vi "Log Data.vi"(8 "error in (no error)":errorcluster, 10 "Data Queue":refnum<queue>, 11 "Logging Configuration":T1={"Log Directory Path"=path "", "Log File Path"=path "", "Log File Prefix"="", "Log File Extension"="", "File Delimiter"=",", "Header Info"=[], "Channels"=[], "Log Instrument Runs"=FALSE}) -> (0 "error out":errorcluster)   [LabVIEW 2020, in "Mock Temperature Controller Control Panel.lvlib" / "Logging.lvlib"]
doc: "This VI uses the TDMS Write function to write data to a TDMS file."
uses:
  Logging.lvlib
  Logging Configuration.ctl
  Instrument Manager/Instrument State.ctl
  <vilib>/Utility/file.llb/Write Delimited Spreadsheet (string).vi
  Instrument Manager/Instrument Manager.lvlib
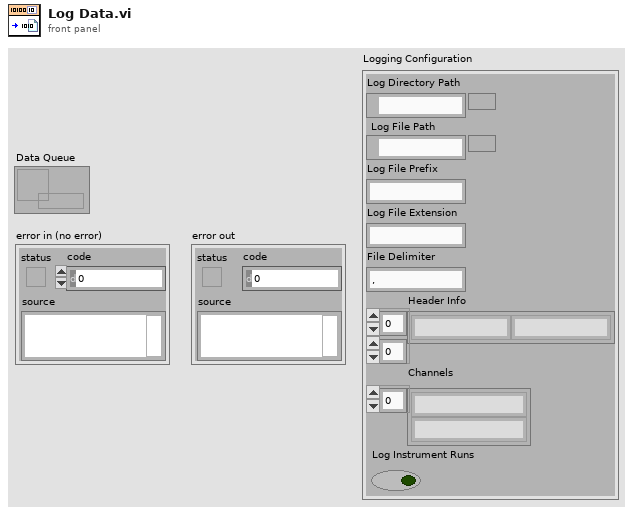
[diagram p1: front panel]
types:
  T1 = typedef "Mock Temperature Controller Control Panel.lvlib/Logging.lvlib/Logging Configuration.ctl" = cluster{"Log Directory Path":path, "Log File Path":path, "Log File Prefix":string, "Log File Extension":string, "File Delimiter":string, "Header Info":string[][], "Channels":string[], "Log Instrument Runs":bool}
  T2 = typedef "Mock Temperature Controller Control Panel.lvlib/Instrument Manager.lvlib/Instrument State.ctl" = cluster{"VISA Resource":refnum<visa-resource-name>, "Setpoint":dbl, "Running":bool, "Running Since":timestamp, "Data Point":cluster{"Time Stamp":timestamp, "Value":dbl}, "Current Temperature":dbl, "Sampling Rate (sec/sample)":dbl}
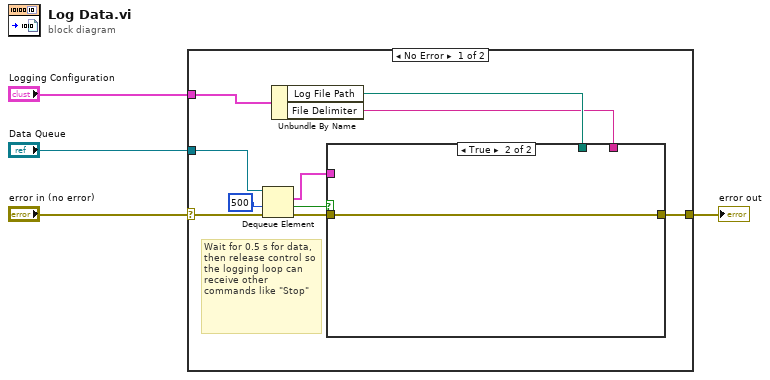
[diagram p0: block diagram]
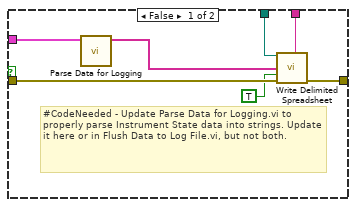
[diagram p2: hidden frame]
diagram:
  n1 = case shown="No Error" "error in (no error)" {
    selector: "error in (no error)" -> [w12 w23]
    tunnel: "Logging Configuration" -> [w14 _]
    tunnel: "Data Queue" -> [w11 _]
    tunnel: [w13 w23] -> w2
    frame No Error {
      # "Wait for 0.5 s for data, then release control so the logging loop can receive other commands like \"Stop\""
      n2 = Dequeue Element(queue=w11, timeout in ms (-1)=500, error in (no error)=w12) -> (element=w8:T2, timed out?=w5:bool, error out=w10:errorcluster)  [unwired: 1 out]
      n3 = Unbundle By Name(w14) -> ("Log File Path"=w9:path, "File Delimiter"=w7:string)
      n4 = case shown="True" w5 {
        tunnel: [w21 w22] -> w13
        tunnel: w10 -> [w20 w22]
        tunnel: w9 -> [w19 _]
        tunnel: w8 -> [w17 _]
        tunnel: w7 -> [w15 _]
        frame False {
          # "#CodeNeeded - Update Parse Data for Logging.vi to properly parse Instrument State data into strings. Update it here or in Flush Data to Log File.vi, but not both."
          n5 = call "Parse Data for Logging.vi"("Instrument State"=w17) -> ("Array"=w16:string[])  [unwired: 10 in]
          n6 = call-poly <vilib>:"Write Delimited Spreadsheet.vi"("file path (dialog if empty)"=w19, "1D data"=w16, "append to file? (new file:F)"=TRUE, "error in (no error)"=w20, "delimiter (\\t)"=w15) -> ("error out"=w21:errorcluster)  [unwired: 9 in, 1 out]
        }
        frame True {
        }
      }
    }
    frame Error {
    }
  }
  "error out" <- w2
